vi "Test 1.vi"() -> ()   [LabVIEW 2016]
uses:
  listbox/listbox.lvclass
  LNK/Copy/Copy.lvclass
  C:/Users/ok/Desktop/camera parameters/ListboxMenu/LNK/Parent Class/Menu.lvclass
  LNK/Delete/Delete.lvclass
  LNK/UP/UP.lvclass
  LNK/Down/Down.lvclass
  LNK/Line/Line.lvclass
  listbox/listbox.lvclass/listbox.ctl
panel:
  out "Row":i32
  out "新值":i32
  in  "停止":bool
  in  "多列列表框":i32(listbox)=4
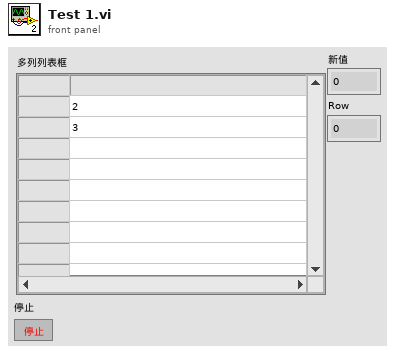
[diagram p1: front panel]
types:
  T1 = typedef "LVPoint32TypeDef.ctl" = cluster{"Horizontal":i32, "Vertical":i32}
  T2 = typedef "LVRowAndColumnTypeDef.ctl" = cluster{"Row":i32, "Column":i32}
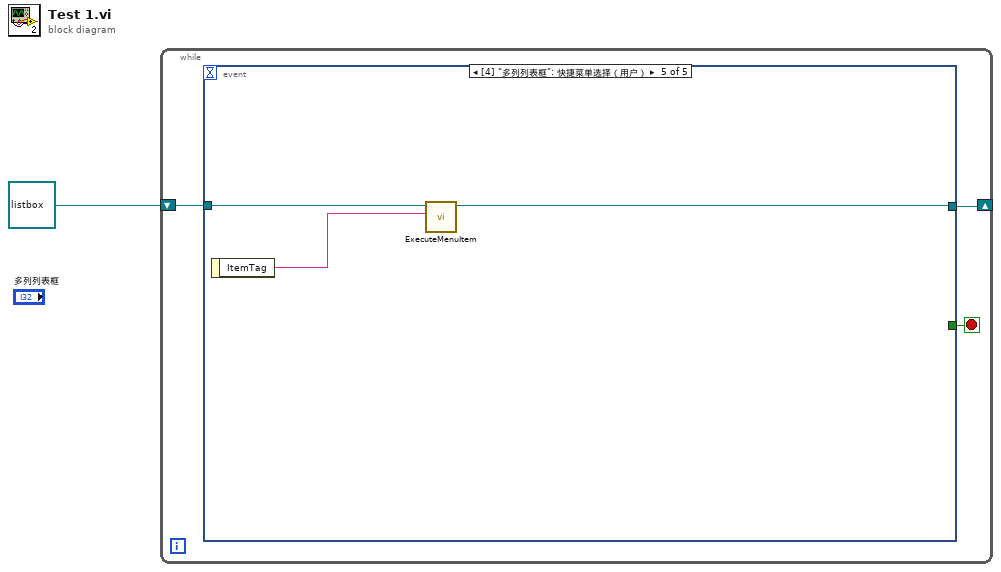
[diagram p0: block diagram]
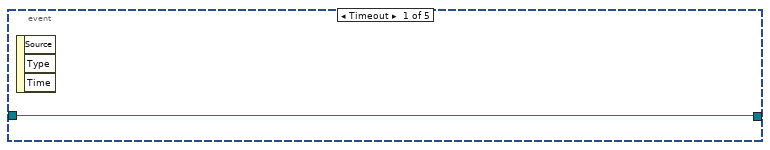
[diagram p2: hidden frame]
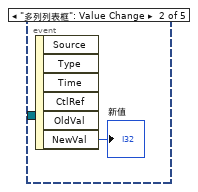
[diagram p3: hidden frame]
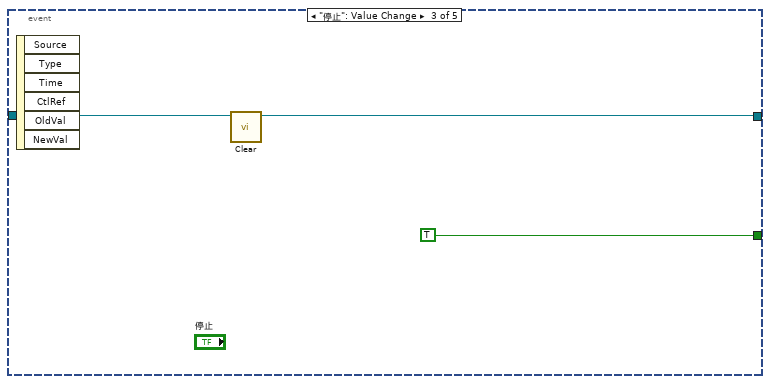
[diagram p4: hidden frame]
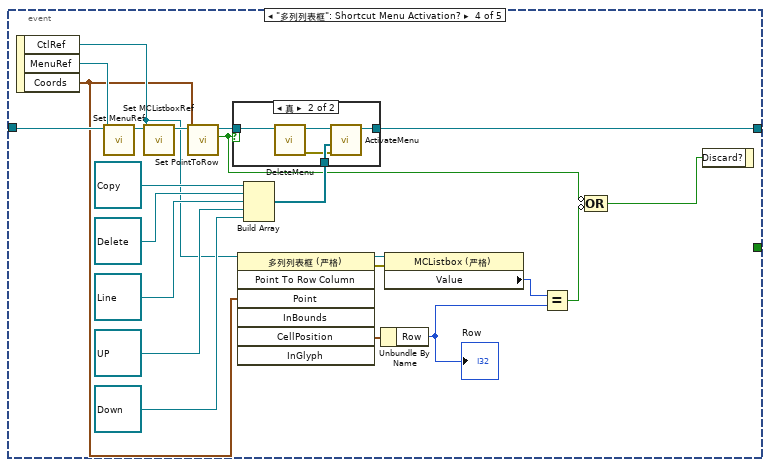
[diagram p5: hidden frame]
diagram:
  n1 = while {
    shift-right: [w2] -> _
    shift-left: refnum<class "listbox.lvclass"> refnum ("listbox.lvclass") -> [w3]
    stop <- w4 stop-if-true
    n2 = event shown="[4] \"多列列表框\": 快捷菜单选择（用户）" {
      selector: _ -> [_ _ _ _ _]
      dyn-events: _ -> [_ _ _ _ _]
      timeout: _ -> [_ _ _ _ _]
      tunnel: [_ _ TRUE _ _] -> w4
      tunnel: w3 -> [w5 _ w8 w31 w40]
      tunnel: [w5 _ w7 w25 w39] -> w2
      event Timeout {
        n3 = event-data() -> ()  [unwired: 1 in, 3 out]
      }
      event "多列列表框": Value Change {
        n4 = event-data() -> ("NewVal"=→"新值":i32)  [unwired: 1 in, 5 out]
      }
      event "停止": Value Change {
        n5 = event-data() -> ()  [unwired: 1 in, 6 out]
        n6 = call "Clear.vi"("listbox 输入"=w8) -> ("listbox 输出"=w7:refnum<class "listbox.lvclass">)  [unwired: 9 in, 1 out]
      }
      event "多列列表框": Shortcut Menu Activation? {
        n7 = event-data() -> ("CtlRef"=w19:refnum<vi>, "MenuRef"=w30:refnum<k9>, "Coords"=w18:T1)  [unwired: 1 in]
        n8 = call "Set MenuRef.vi"("MenuRef"=w30, "listbox in"=w31) -> ("listbox out"=w29:refnum<class "listbox.lvclass">)  [unwired: 9 in]
        n9 = call "Set MCListboxRef.vi"("MCListboxRef"=w19, "listbox in"=w29) -> ("listbox out"=w28:refnum<class "listbox.lvclass">)  [unwired: 9 in]
        n10 = call "Set PointToRow.vi"("坐标"=w18, "listbox 输入"=w28) -> ("边界内？"=w11:bool, "listbox 输出"=w24:refnum<class "listbox.lvclass">)  [unwired: 7 in, 1 out]
        n11 = invoke class="多列列表框 (严格)" method="Point To Row Column"(reference=w19, "Point"=w18) -> (reference out=w16:refnum<vi>, error out=w15:errorcluster, "CellPosition"=w17:T2)  [unwired: 5 in, 4 out]
        n12 = Build Array(refnum<class "Copy.lvclass"> refnum ("Copy.lvclass"), refnum<class "Delete.lvclass"> refnum ("Delete.lvclass"), refnum<class "Line.lvclass"> refnum ("Line.lvclass"), refnum<class "UP.lvclass"> refnum ("UP.lvclass"), refnum<class "Down.lvclass"> refnum ("Down.lvclass")) -> (w26:refnum<class "Menu.lvclass">[])
        n13 = case shown="真" w11 {
          tunnel: w26 -> [_ w37]
          tunnel: [w32 w36] -> w25
          tunnel: w24 -> [w32 w33]
          frame False {
          }
          frame True {
            n14 = call "DeleteMenu.vi"("listbox 输入"=w33) -> ("error out"=w34:errorcluster, "listbox 输出"=w35:refnum<class "listbox.lvclass">)  [unwired: 9 in]
            n15 = call "ActivateMenu.vi"("error in (no error)"=w34, "MenuClassArray"=w37, "listbox 输入"=w35) -> ("listbox 输出"=w36:refnum<class "listbox.lvclass">)  [unwired: 7 in, 1 out]
          }
        }
        n16 = Unbundle By Name(w17) -> ("Row"=w13:i32)
        "Row" <- w13
        n17 = property class="MCListbox (严格)"(reference=w16, error in=w15) -> ("Value"=w14:i32)  [unwired: 2 out]
        n18 = Equal?(x=w14, y=w13) -> (x = y?=w12:bool)
        n19 = Compound Arithmetic op=OR ("复合运算")(invert w11, invert w12) -> (w10:bool)
        n20 = event-data("Discard?"=w10) -> ()  [unwired: 1 in, 1 out]
      }
      event "多列列表框": Shortcut Menu Selection (User) {
        n21 = event-data() -> ("ItemTag"=w38:string)  [unwired: 1 in]
        n22 = call "ExecuteMenuItem.vi"("项标识符"=w38, "listbox 输入"=w40) -> ("listbox 输出"=w39:refnum<class "listbox.lvclass">)  [unwired: 8 in, 1 out]
      }
    }
  }
